vi "test Source.vi"(8 "error in (no error)":errorcluster, 11 "TestCase in":refnum<class "Parameter Setting.lvclass">) -> (0 "error out":errorcluster, 3 "TestCase out":refnum<class "Parameter Setting.lvclass">)   [LabVIEW 2017, in "Deterministic Error Tests.lvlib" / "Parameter Setting.lvclass"]
uses:
  Parameter Setting.lvclass
  Parameter Setting.lvclass/Parameter Setting.ctl
  <vilib>/addons/_JKI Toolkits/VI Tester/TestCase.llb/TestCase.lvclass
  Source/Deterministic Error Builder.lvlib
  C:/Program Files (x86)/National Instruments/LabVIEW 2017/vi.lib/addons/_JKI Toolkits/VI Tester/TestCase.llb/TestCase.lvclass
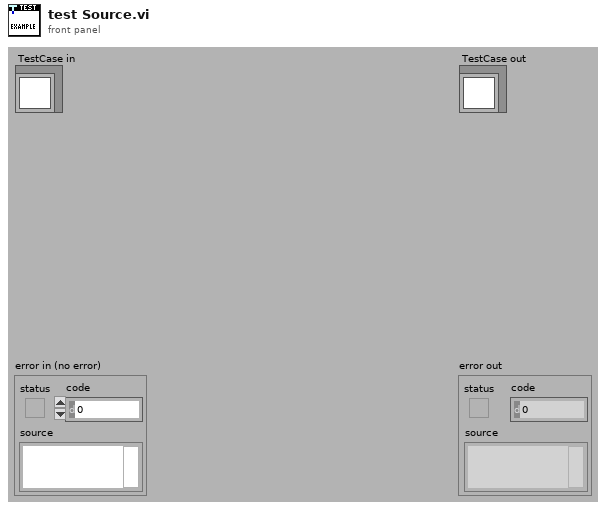
[diagram p1: front panel]
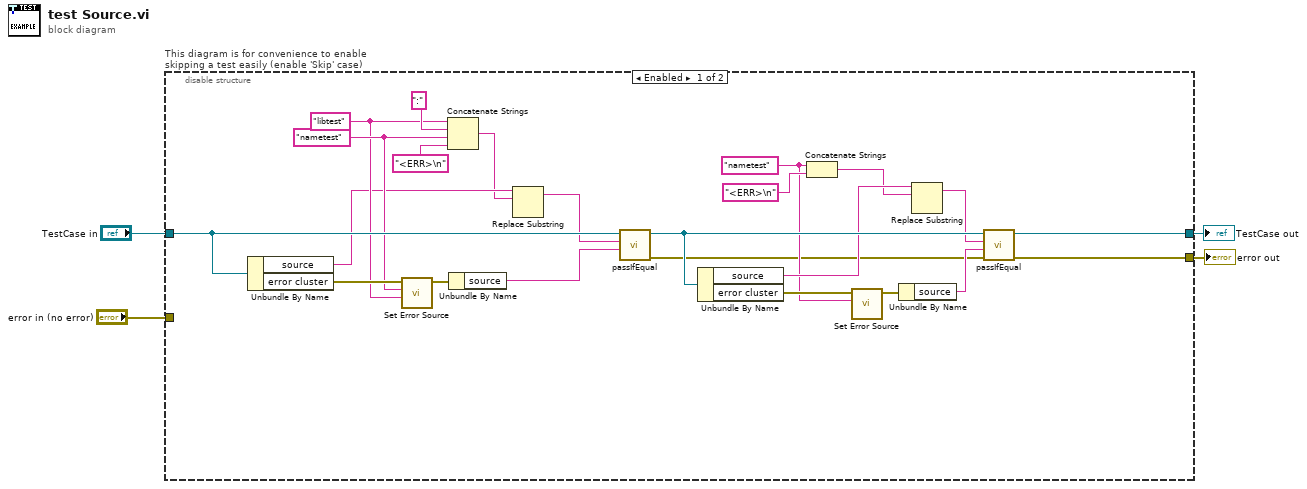
[diagram p0: block diagram]
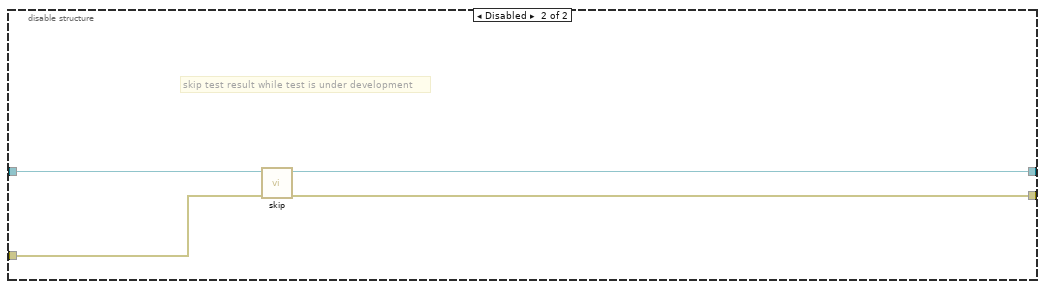
[diagram p2: hidden frame]
diagram:
  n1 = disable-structure "This diagram is for convenience to enable skipping a test easily (enable 'Skip' case)" shown="Enabled" {
    disable-tunnel: "TestCase in" -> [w27 w31]
    disable-tunnel: [w16 w29] -> w2
    disable-tunnel: [w8 w30] -> w1
    disable-tunnel: "error in (no error)" -> [_ w28]
    frame Enabled {
      w9 = "nametest"
      w21 = "nametest"
      w20 = "libtest"
      n2 = Unbundle By Name(w27) -> ("source"=w19:string, "error cluster"=w25:errorcluster)
      n3 = call "Set Error Source.vi"("library name (\"\")"=w20, "vi name"=w21, "error in"=w25) -> ("error out"=w24:errorcluster)  [unwired: 7 in, 1 out]
      n4 = Concatenate Strings(w20, ":" ("string"), w21, "<ERR>\n") -> (w17:string)
      n5 = Unbundle By Name(w24) -> ("source"=w26:string)
      n6 = Replace Substring(4:w17, 5:w19) -> (1:w18:string)  [unwired: 2 in, 1 out]
      n7 = call-dynamic "passIfEqual.vi"("y"=w26, "x"=w18, "TestCase in"=w27) -> ("error out"=w7:errorcluster, "TestCase out"=w13:refnum<class "Parameter Setting.lvclass">)  [unwired: 7 in]
      n8 = Unbundle By Name(w13) -> ("source"=w10:string, "error cluster"=w14:errorcluster)
      n9 = Concatenate Strings(w9, "<ERR>\n") -> (w6:string)
      n10 = call "Set Error Source.vi"("vi name"=w9, "error in"=w14) -> ("error out"=w15:errorcluster)  [unwired: 8 in, 1 out]
      n11 = Unbundle By Name(w15) -> ("source"=w12:string)
      n12 = Replace Substring(4:w6, 5:w10) -> (1:w5:string)  [unwired: 2 in, 1 out]
      n13 = call-dynamic "passIfEqual.vi"("error in (no error)"=w7, "y"=w12, "x"=w5, "TestCase in"=w13) -> ("error out"=w8:errorcluster, "TestCase out"=w16:refnum<class "Parameter Setting.lvclass">)  [unwired: 6 in]
    }
    frame Disabled {
      # "skip test result while test is under development"
      n14 = call <vilib>:"skip.vi"("error in (no error)"=w28, "TestCase in"=w31) -> ("error out"=w30:errorcluster, "TestCase out"=w29:refnum<class "Parameter Setting.lvclass">)  [unwired: 8 in]
    }
  }
  "error out" <- w1
  "TestCase out" <- w2
